vi "Split Deckblatt Table.vi"(9 "Deckblatt":bool, 10 "Array (Eingang)":T1[][](array[typedef]), 11 "Numbre of Rows for TitlePage":i32) -> (2 "HeaderTable":T1[][](array[typedef]), 3 "TitlePage_HeaderTable":T1[][](array[typedef]))   [LabVIEW 2020, in "Linearisierung v2.lvlib" / "Protokoll.lvlib"]
uses:
  Protokoll.lvlib
  Visualisierungs Elemente/String - Ausgabefeld.ctl
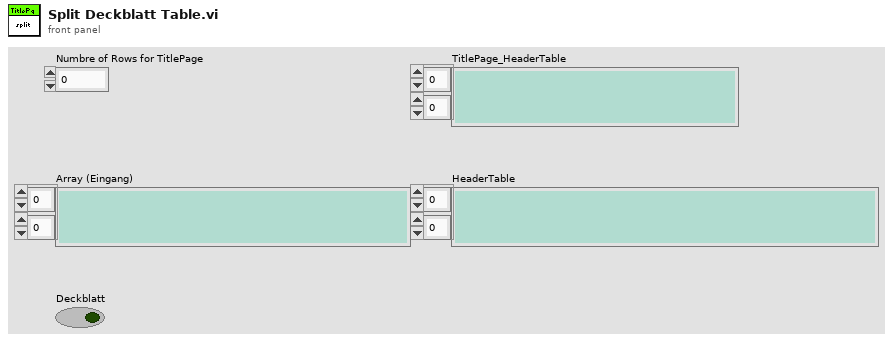
[diagram p1: front panel]
types:
  T1 = typedef "String - Ausgabefeld.ctl" = string
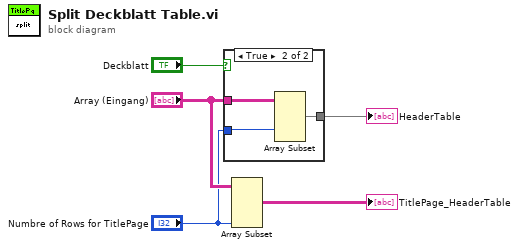
[diagram p0: block diagram]
diagram:
  n1 = case shown="True" "Deckblatt" {
    tunnel: "Array (Eingang)" -> [w6 w9]
    tunnel: "Numbre of Rows for TitlePage" -> [_ w7]
    tunnel: [w6 w8] -> w4
    frame False {
    }
    frame True {
      n2 = Array Subset(array=w9, index (col)=w7) -> (w8:T1[][])  [unwired: 3 in]
    }
  }
  "HeaderTable" <- w4
  n3 = Array Subset(array="Array (Eingang)", length (col)="Numbre of Rows for TitlePage") -> (→"TitlePage_HeaderTable":T1[][])  [unwired: 3 in]
